vi "Event Logger.vi"(5 "Event Name":string, 7 "Event Description":string, 11 "Error in (no error)":errorcluster, 13 "Operation":T1(ring)=enum."Close Event Log") -> (15 "Error out":errorcluster)   [LabVIEW 2022 SP3]
uses:
  <vilib>/NI/Event Logger Library/EventLog/EventLog.lvclass
  <vilib>/NI/Event Logger Library/EventLog/Initialize_TDMS.vi
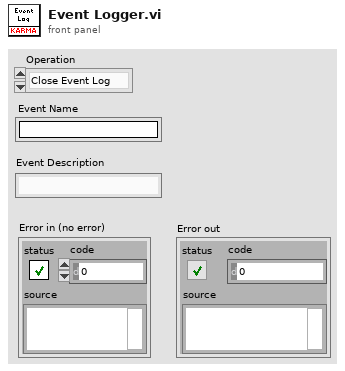
[diagram p1: front panel]
types:
  T1 = enum16{"Initialize", "Log Events", "Close Event Log"}
  T2 = typedef "Paths.ctl" = cluster{"Configuration":path, "Event Logs":path, "Error Logs":path, "Configuration.ini":path}
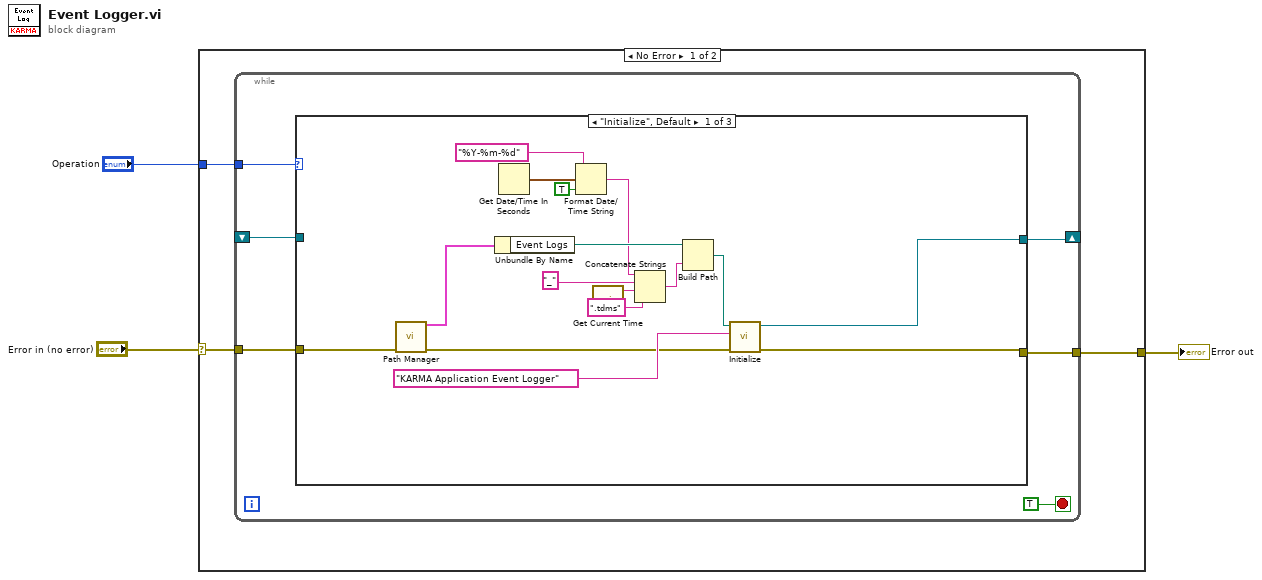
[diagram p0: block diagram]
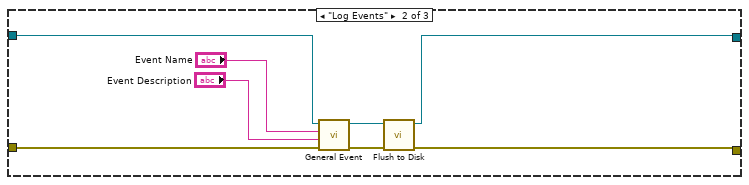
[diagram p2: hidden frame]
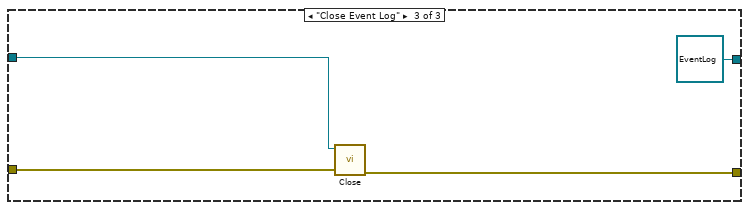
[diagram p3: hidden frame]
diagram:
  n1 = case shown="No Error" "Error in (no error)" {
    selector: "Error in (no error)" -> [w5 w41]
    tunnel: "Operation" -> [w6 _]
    tunnel: [w4 w41] -> w1
    frame No Error {
      n2 = while {
        tunnel: w6 -> [w12]
        tunnel: w5 -> [w11]
        shift-right: [w10] -> _
        shift-left: _ -> [w9]
        tunnel: [w8] -> w4
        stop <- TRUE stop-if-true
        n3 = case shown="\"Initialize\", Default" w12 {
          tunnel: w11 -> [w21 w34 w40]
          tunnel: [w22 w32 refnum<class "EventLog.lvclass"> refnum ("EventLog ref")] -> w10
          tunnel: w9 -> [_ w33 w39]
          tunnel: [w17 w29 w37] -> w8
          frame "Initialize", Default {
            n4 = call "Path Manager.vi"("error in (no error)"=w21) -> ("Cluster"=w19:T2, "Error out"=w20:errorcluster)  [unwired: 13 in]
            n5 = Unbundle By Name(w19) -> ("Event Logs"=w18:path)
            n6 = Get Date/Time In Seconds() -> (seconds since 1Jan1904=w14:timestamp)
            n7 = Format Date/Time String(time format string (%c)="%Y-%m-%d", seconds (now)=w14, UTC format=TRUE) -> (date/time string=w13:string)
            n8 = call "Get Current Time.vi"() -> ("Time String"=w26:string)  [unwired: 8 in]
            n9 = Concatenate Strings(w13, "_" ("string"), w26, ".tdms" ("string")) -> (w27:string)
            n10 = Build Path(base path=w18, name or relative path=w27) -> (appended path=w28:path)
            n11 = call-poly <vilib>:"Initialize.vi"("error in (no error)"=w20, "Description"="KARMA Application Event Logger", "Path"=w28) -> ("error out"=w17:errorcluster, "EventLog ref"=w22:refnum<class "EventLog.lvclass">)  [unwired: 7 in]
          }
          frame "Log Events" {
            n12 = call <vilib>:"General Event.vi"("error in (no error)"=w34, "Event Description"="Event Description", "Event Name"="Event Name", "EventLog ref"=w33) -> ("error out"=w35:errorcluster, "EventLog ref"=w36:refnum<class "EventLog.lvclass">)  [unwired: 6 in]
            n13 = call <vilib>:"Flush to Disk.vi"("error in (no error)"=w35, "EventLog ref"=w36) -> ("error out"=w29:errorcluster, "EventLog ref"=w32:refnum<class "EventLog.lvclass">)  [unwired: 8 in]
          }
          frame "Close Event Log" {
            n14 = call <vilib>:"Close.vi"("error in (no error)"=w40, "EventLog ref"=w39) -> ("error out"=w37:errorcluster)  [unwired: 9 in]
          }
        }
      }
    }
    frame Error {
    }
  }
  "Error out" <- w1
